vi "Drive Straight.vi"(2 "Max Power":dbl=0.35 format="%#_13g", 3 "output range":cluster{"output high":dbl, "output low":dbl}={"output high"=1.0, "output low"=-1.0} {"output low" format="%.2f"; "output high" format="%.2f"}, 5 "Swerve DevRef":T2[](array[typedef]), 6 "Wheel DevRef":T2[](array[typedef]), 7 "Drive Angle":dbl=3.141592653589793, 9 "Time Condition":u32=10000, 11 "Total Distance( ticks )":dbl format="%#_13g", 12 "Start Power":dbl format="%#_13g", 13 "Min Power":dbl=0.35 format="%#_13g", 14 "PID gains Rotational Correction":T1={"proportional gain (Kc)"=0.0001, "integral time (Ti, min)"=0.0, "derivative time (Td, min)"=0.0} {"derivative time (Td, min)" format="%.3f"; "integral time (Ti, min)" format="%.6f"; "proportional gain (Kc)" format="%.9f"}, 15 "error in":errorcluster) -> (4 "error out":errorcluster)   [LabVIEW 2017, in "Huskie Swerve.lvlib"]
uses:
  Huskie Swerve.lvlib
  <vilib>/Analysis/NI_AALBase.lvlib
  <vilib>/Analysis/baseanly.llb/Mean (DBL).vi
  <vilib>/addons/control/pid/NI_PID_pid.lvlib
  <vilib>/addons/control/pid/pid.llb/PID (DBL).vi
  Public/Documents/Cross The Road Electronics/Phoenix-LabVIEW/Motor Controller/Get/CTRE_Phoenix_MotorController_GetSelectedSensorData.vi
  <vilib>/Rock Robotics/SystemInterfaces/DIO/FPGA_DIOPWMChannel.ctl
  <vilib>/Rock Robotics/WPI/PWM/WPI_PWMDeadband.ctl
  <vilib>/Rock Robotics/WPI/MotorControl/WPI_MotorControlType.ctl
  <vilib>/Rock Robotics/WPI/MotorControl/WPI_MotorControlDeviceRef.ctl
  <vilib>/Rock Robotics/SystemInterfaces/DIO/FPGA_DIOChannel.ctl
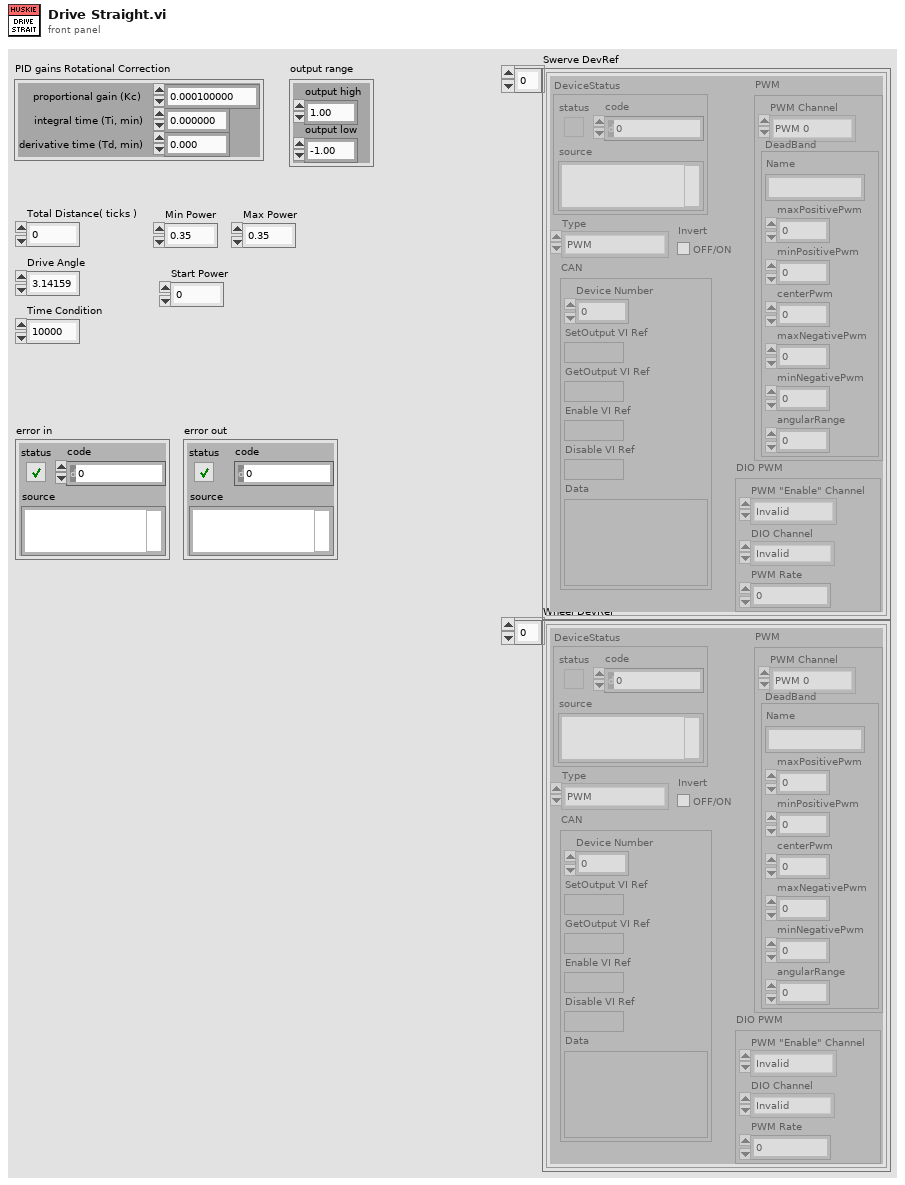
[diagram p1: front panel]
types:
  T1 = cluster{"proportional gain (Kc)":dbl, "integral time (Ti, min)":dbl, "derivative time (Td, min)":dbl}
  T2 = typedef "WPI_MotorControlDeviceRef.ctl" = cluster{"DeviceStatus":errorcluster, "Type":T3, "PWM":cluster{"PWM Channel":T4, "DeadBand":T5}, "CAN":cluster{"Device Number":u8, "SetOutput VI Ref":variant, "GetOutput VI Ref":variant, "Enable VI Ref":variant, "Disable VI Ref":variant, "Data":variant}, "Invert":bool, "DIO PWM":cluster{"PWM \"Enable\" Channel":T4, "DIOChannel":T6, "PWM Rate":dbl}}
  T3 = typedef "WPI_MotorControlType.ctl" = enum16{"PWM", "CAN", "DIO PWM"}
  T4 = typedef "FPGA_DIOPWMChannel.ctl" = enum8{"PWM 0", "PWM 1", "PWM 2", "PWM 3", "PWM 4", "PWM 5", "PWM 6", "PWM 7", "PWM 8", "PWM 9", "PWM MXP 0", "PWM MXP 1", "PWM MXP 2", "PWM MXP 3", "PWM MXP 4", "PWM MXP 5", "PWM MXP 6", "PWM MXP 7", "PWM MXP 8", "PWM MXP 9", "Invalid"}
  T5 = typedef "WPI_PWMDeadband.ctl" = cluster{"Name":string, "maxPositivePwm":i32, "minPositivePwm":i32, "centerPwm":i32, "maxNegativePwm":i32, "minNegativePwm":i32, "angularRange":u16}
  T6 = typedef "FPGA_DIOChannel.ctl" = enum8{"DIO 0", "DIO 1", "DIO 2", "DIO 3", "DIO 4", "DIO 5", "DIO 6", "DIO 7", "DIO 8", "DIO 9", "DIO MXP 0", "DIO MXP 1", "DIO MXP 2", "DIO MXP 3", "DIO MXP 4", "DIO MXP 5", "DIO MXP 6", "DIO MXP 7", "DIO MXP 8", "DIO MXP 9", "DIO MXP 10", "DIO MXP 11", "DIO MXP 12", "DIO MXP 13", "DIO MXP 14", "DIO MXP 15", "SPI Port CS1", "SPI Port CS2", "SPI Port CS3", "SPI Port MISO", "SPI Port MOSI", "Invalid"}
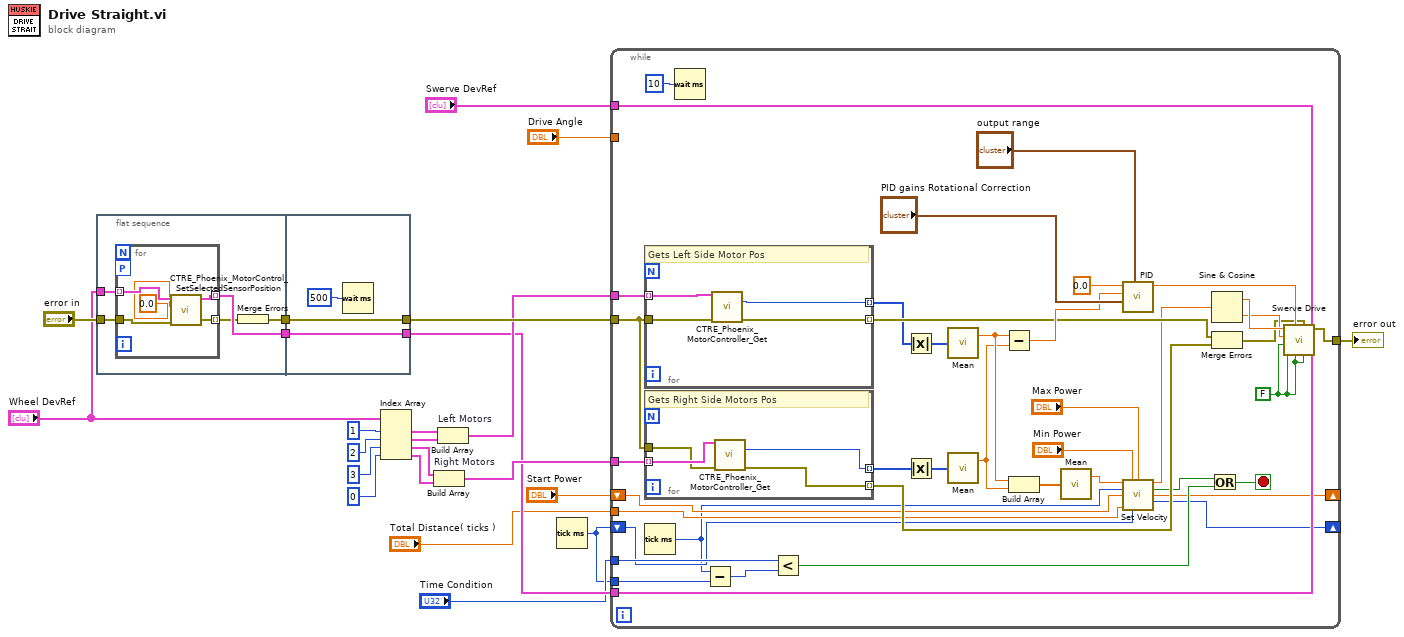
[diagram p0: block diagram]
diagram:
  n1 = flat-sequence {
    tunnel: "Wheel DevRef" -> [w28]
    tunnel: "error in" -> [w26]
    tunnel: [w27] -> w23
    tunnel: [w24] -> w22
    tunnel: [w36] -> w6
    tunnel: w23 -> [w36]
    tunnel: w22 -> [w34]
    tunnel: [w34] -> w11
    frame #0 {
      n2 = for {
        tunnel: w28 -> [w33] mode=indexing
        tunnel: [w31] -> w27 mode=indexing
        workers-P: _ -> [_]
        tunnel: w26 -> [w30]
        tunnel: [w29] -> w25 mode=indexing
        n3 = call "CTRE_Phoenix_MotorControl_SetSelectedSensorPosition.vi"("error in (no error)"=w30, "New Sensor Position"=0.0, "PhoenixMotorControlDevRef"=w33) -> ("error out"=w29:errorcluster, "PhoenixMotorControlDevRef"=w31:T2)  [unwired: 7 in]
      }
      n4 = Merge Errors(w25) -> (w24:errorcluster)
    }
    frame #1 {
      n5 = Wait (ms)(milliseconds to wait=u32 500) -> ()  [unwired: 1 out]
    }
  }
  n6 = Index Array(array="Wheel DevRef", index #1=1 ("index"), index #2=2 ("index"), index #3=3 ("index"), index #4=0 ("index")) -> (element #1=w15:T2, element #2=w16:T2, element #3=w13:T2, element #4=w14:T2)
  n7 = Build Array "Right Motors"(w13, w14) -> (w9:T2[])
  n8 = Build Array "Left Motors"(w15, w16) -> (w10:T2[])
  n9 = Tick Count (ms)() -> (millisecond timer value=w4:u32)
  n10 = while {
    tunnel: w11 -> [w70]
    tunnel: w10 -> [w77]
    tunnel: w9 -> [w76]
    tunnel: "Drive Angle" -> [_]
    tunnel: "Swerve DevRef" -> [w63]
    tunnel: w6 -> [w62]
    tunnel: "Time Condition" -> [w59]
    tunnel: w4 -> [w60]
    shift-right: [w55] -> _
    shift-left: "Start Power" -> [w54]
    shift-right: [w47] -> _
    shift-left: w4 -> [w44]
    tunnel: "Total Distance( ticks )" -> [w45]
    tunnel: [w38] -> w1
    stop <- w57 stop-if-true
    w37 = FALSE ("Straight Drive")
    n11 = for {
      tunnel: [w85] -> w53 mode=indexing
      tunnel: w77 -> [w82] mode=indexing
      tunnel: w70 -> [w83]
      tunnel: [w84] -> w66 mode=indexing
      # "Gets Left Side Motor Pos"
      n12 = call-poly "CTRE_Phoenix_MotorController_Get.vi"("PhoenixMotorControlDevRef"=w82, "error in"=w83) -> ("Position (Raw Sensor Units)"=w85:i32, "error out"=w84:errorcluster)  [unwired: 10 in, 2 out]
    }
    n13 = for {
      tunnel: [w78] -> w52 mode=indexing
      tunnel: w76 -> [w81] mode=indexing
      tunnel: w70 -> [w80]
      tunnel: [w79] -> w65 mode=indexing
      # "Gets Right Side Motors Pos"
      n14 = call-poly "CTRE_Phoenix_MotorController_Get.vi"("PhoenixMotorControlDevRef"=w81, "error in"=w80) -> ("Position (Raw Sensor Units)"=w78:i32, "error out"=w79:errorcluster)  [unwired: 10 in, 2 out]
    }
    n15 = Tick Count (ms)() -> (millisecond timer value=w43:u32)
    n16 = Wait (ms)(milliseconds to wait=u32 10) -> ()  [unwired: 1 out]
    n17 = Subtract(x=w43, y=w60) -> (x-y=w61:u32)
    n18 = Less?(x=w59, y=w61) -> (x < y?=w58:bool)
    n19 = Absolute Value(x=w53) -> (abs(x)=w42:i32[])
    n20 = Absolute Value(x=w52) -> (abs(x)=w41:i32[])
    n21 = call-poly <vilib>:"Mean.vi"("X"=w42) -> ("mean"=w51:dbl)  [unwired: 1 out]
    n22 = call-poly <vilib>:"Mean.vi"("X"=w41) -> ("mean"=w50:dbl)  [unwired: 1 out]
    n23 = Subtract(x=w51, y=w50) -> (x-y=w71:dbl)
    n24 = Build Array(w51, w50) -> (w49:dbl[])
    n25 = call-poly <vilib>:"Mean.vi"("X"=w49) -> ("mean"=w48:dbl)  [unwired: 1 out]
    n26 = call-poly <vilib>:"PID.vi"("output range"="output range", "PID gains"="PID gains Rotational Correction", "process variable"=w71, "setpoint"=0.0) -> ("output"=w67:dbl)  [unwired: 6 in, 1 out]
    n27 = call "Set Velocity.vi"("Process Variable(x)"=w48, "Min Power"="Min Power", "Max Power"="Max Power", "Current TIme"=w43, "Current Power"=w54, "Total Distance"=w45, "Last Time Input"=w44) -> ("Coerced Motor power"=w46:dbl, "End Loop?"=w56:bool, "Non-Coerced Motor Power"=w55:dbl, "Last Time Output"=w47:u32)  [unwired: 5 in]
    n28 = Or(x=w56, y=w58) -> (x .or. y?=w57:bool)
    n29 = Sine & Cosine(0:w46) -> (1:w69:dbl, 2:w68:dbl)
    n30 = Merge Errors(w66, w65) -> (w64:errorcluster)
    n31 = call "Swerve Drive.vi"("Drive Dev Ref"=w62, "Swerve Dev Ref"=w63, "X Drive"=w37, "error in"=w64, "Low Sensitivity"=w37, "Z"=w67, "Reverse Drive"=w37, "Straight Drive"=w37, "Y"=w68, "X"=w69) -> ("error out"=w38:errorcluster)  [unwired: 1 in]
  }
  "error out" <- w1
